vi "33250A_control.vi"() -> ()   [LabVIEW 2019]
uses:
  <userlib>/_TI-LA/Instr Drivers/Signal Generator/33XXX/Driver/EasyIO/Typedef/33XXX Standard Waveform Configuration.ctl
  <userlib>/_TI-LA/Instr Drivers/Signal Generator/33XXX/Driver/EasyIO/Typedef/33XXX Waveform Function.ctl
  <userlib>/_TI-LA/Instr Drivers/Signal Generator/33XXX/Driver/EasyIO/Typedef/33XXX Waveform Unit.ctl
  <userlib>/_TI-LA/Instr Drivers/Signal Generator/33XXX/Driver/EasyIO/Typedef/33XXX Output Load.ctl
  <userlib>/_TI-LA/Instr Drivers/Signal Generator/33XXX/Driver/EasyIO/Typedef/33XXX Output Load Termination.ctl
  <userlib>/_TI-LA/Instr Drivers/Signal Generator/33XXX/Modules/33XXX Modules.lvlib
  <userlib>/_TI-LA/Instr Drivers/Signal Generator/33XXX/Driver/33XXX.lvlib
panel:
  in  "Enable Output?":bool=TRUE
  in  "Standard Waveform Configuration":T1={"Frequency (Hz)"=1000.0, "Waveform Function"=1, "DC Offset (V)"=0.0, "Unit"=0, "Amplitude (V)"=1.0, "Duty cycle (%)"=50.0} {"Duty cycle (%)" min=0.002 max=99.999 step=0.001 format="%.3p"; "Amplitude (V)" min=0.001 max=20.0 format="%#_6p"; "Unit" items=["Vpp", "Vrms", "dB"]; "DC Offset (V)" min=-10.0 max=10.0 format="%#_6p"; "Waveform Function" items=["DC", "Sine", "Square", "Triangle", "Ramp", "Pulse", "Noise", "Sinc", "Negative Ramp", "Exponential Rise", "Exponential Fall", "Cardiac"]; "Frequency (Hz)" min=1e-06 max=80000000.0 format="%#_6p"}
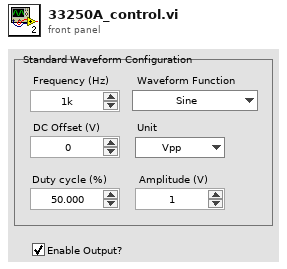
[diagram p1: front panel]
types:
  T1 = typedef "33XXX.lvlib/33XXX Standard Waveform Configuration.ctl" = cluster{"Frequency (Hz)":dbl, "Waveform Function":T2, "DC Offset (V)":dbl, "Unit":T3, "Amplitude (V)":dbl, "Duty cycle (%)":dbl}
  T2 = typedef "33XXX.lvlib/33XXX Waveform Function.ctl" = u16
  T3 = typedef "33XXX.lvlib/33XXX Waveform Unit.ctl" = u16
  T4 = typedef "33XXX.lvlib/33XXX Output Load.ctl" = cluster{"Output Load Impedence":T5, "Load value (ohms)":dbl}
  T5 = typedef "33XXX.lvlib/33XXX Output Load Termination.ctl" = enum16{"50 Ohms", "High Z", "User Defined"}
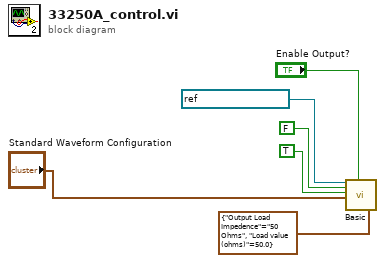
[diagram p0: block diagram]
diagram:
  n1 = call <userlib>:"Basic.vi"("Instrument Address"=refnum<visa-resource-name> "GPIB0::3::INSTR", "Reset?"=FALSE, "ID Query?"=TRUE, "Standard Waveform Configuration"="Standard Waveform Configuration", "Enable Output?"="Enable Output?", "Output Load Configuration"=T4 {"Output Load Impedence"=enum."50 Ohms", "Load value (ohms)"=50.0}) -> ()  [unwired: 11 in, 3 out]
